vi "storage.vi"(2 "Dataflow In #2":errorcluster, 3 "Dataflow In #3":errorcluster, 4 "Dataflow In #1":errorcluster) -> (1 "Dataflow Out":errorcluster)   [LabVIEW 2019]
uses:
  lib/libSimulationControl/libSimulationControl.lvlib
panel:
  # "*******************************************************************\nBiogas Plant Control\n\nAuthor: Paul Zügel\nGCSC-Frankfurt am Main 2020\n\n*******************************************************************"
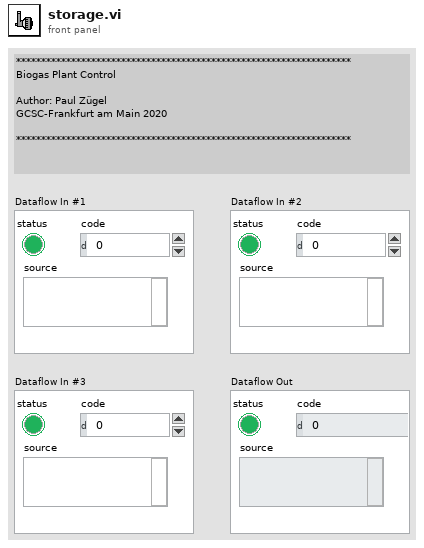
[diagram p1: front panel]
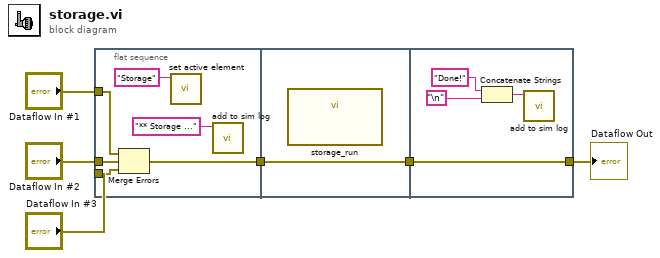
[diagram p0: block diagram]
diagram:
  n1 = flat-sequence {
    tunnel: "Dataflow In #1" -> [w12]
    tunnel: "Dataflow In #2" -> [w11]
    tunnel: "Dataflow In #3" -> [w10]
    tunnel: [w9] -> w2
    tunnel: [w13] -> w3
    tunnel: w2 -> [w13]
    tunnel: [w17] -> w1
    tunnel: w3 -> [w17]
    frame #0 {
      n2 = Merge Errors(w12, w11, w10) -> (w9:errorcluster)
      n3 = call "set active element.vi"("elem"="Storage") -> ()  [unwired: 10 in, 1 out]
      n4 = call "add to sim log.vi"("log"="** Storage ..." ("string")) -> ()  [unwired: 10 in, 1 out]
    }
    frame #1 {
      n5 = call "storage_run.vi"() -> ()  [unwired: 12 in]
    }
    frame #2 {
      n6 = Concatenate Strings("Done!" ("string"), "\n") -> (w14:string)
      n7 = call "add to sim log.vi"("log"=w14) -> ()  [unwired: 10 in, 1 out]
    }
  }
  "Dataflow Out" <- w1
